vi "matrici_v0.vi"() -> ()   [LabVIEW 2009]
panel:
  in  "stop":bool
  out "Waveform Graph":dbl[](graph)=[1.8551209897835594, 0.4969141781827492, 9.634163186118114, 0.7662289420876345, 5.001697647029765, 10.090204060892423, 3.6408733534201123, 1.373703936255532, 0.023268686246756154, 7.321341021440192, 4.073774868622181, 10.508838182739613]
  in  "Valoarea maxima":dbl(knob)=10.969341767682025 scale=0.0..100.0
  out "Array":dbl[](array[numeric])=[1.8551209897835594, 0.4969141781827492, 9.634163186118114, 0.7662289420876345, 5.001697647029765, 10.090204060892423, 3.6408733534201123, 1.373703936255532, 0.023268686246756154, 7.321341021440192, 4.073774868622181, 10.508838182739613]
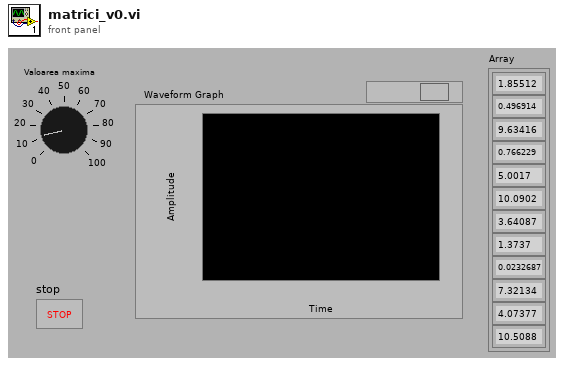
[diagram p1: front panel]
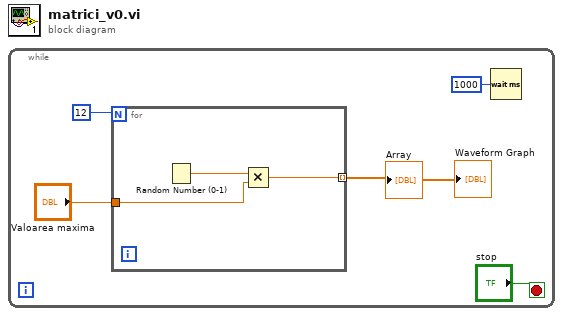
[diagram p0: block diagram]
diagram:
  n1 = while {
    stop <- "stop" stop-if-true
    n2 = for {
      N: 12 -> [_]
      tunnel: [w7] -> w3 mode=indexing
      tunnel: "Valoarea maxima" -> [w6]
      n3 = Random Number (0-1)() -> (number: 0 to 1=w8:dbl)
      n4 = Multiply(x=w8, y=w6) -> (x*y=w7:dbl)
    }
    "Array" <- w3
    "Waveform Graph" <- w3
    n5 = Wait (ms)(milliseconds to wait=u32 1000) -> ()  [unwired: 1 out]
  }
